vi "mixer.vi"(6 "Ready For Output":bool, 8 "Input Valid":bool, 9 "cos":fxp<+/-,16,2>, 10 "sin":fxp<+/-,16,2>, 11 "AI":fxp<+/-,16,1>) -> (0 "Output Valid":bool, 2 "Y":fxp<+/-,20,2> format="%.19g", 3 "X":fxp<+/-,20,2> format="%.19g", 4 "Ready For Input":bool=TRUE)   [LabVIEW 2018, in "SCTL.lvlib"]
doc: "This VI is used in four wire handshake."
uses:
  SCTL.lvlib
  <vilib>/rvi/FXPMathLib/FxpMul/XNode/nifxpmath_Multiplier.xnode
  <vilib>/rvi/FXPMathLib/sim/FxpSim.dll
panel:
  # "Inputs"
  # "Outputs"
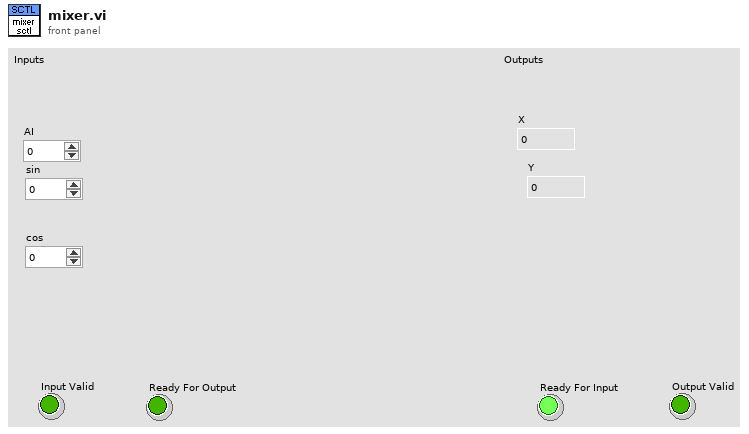
[diagram p1: front panel]
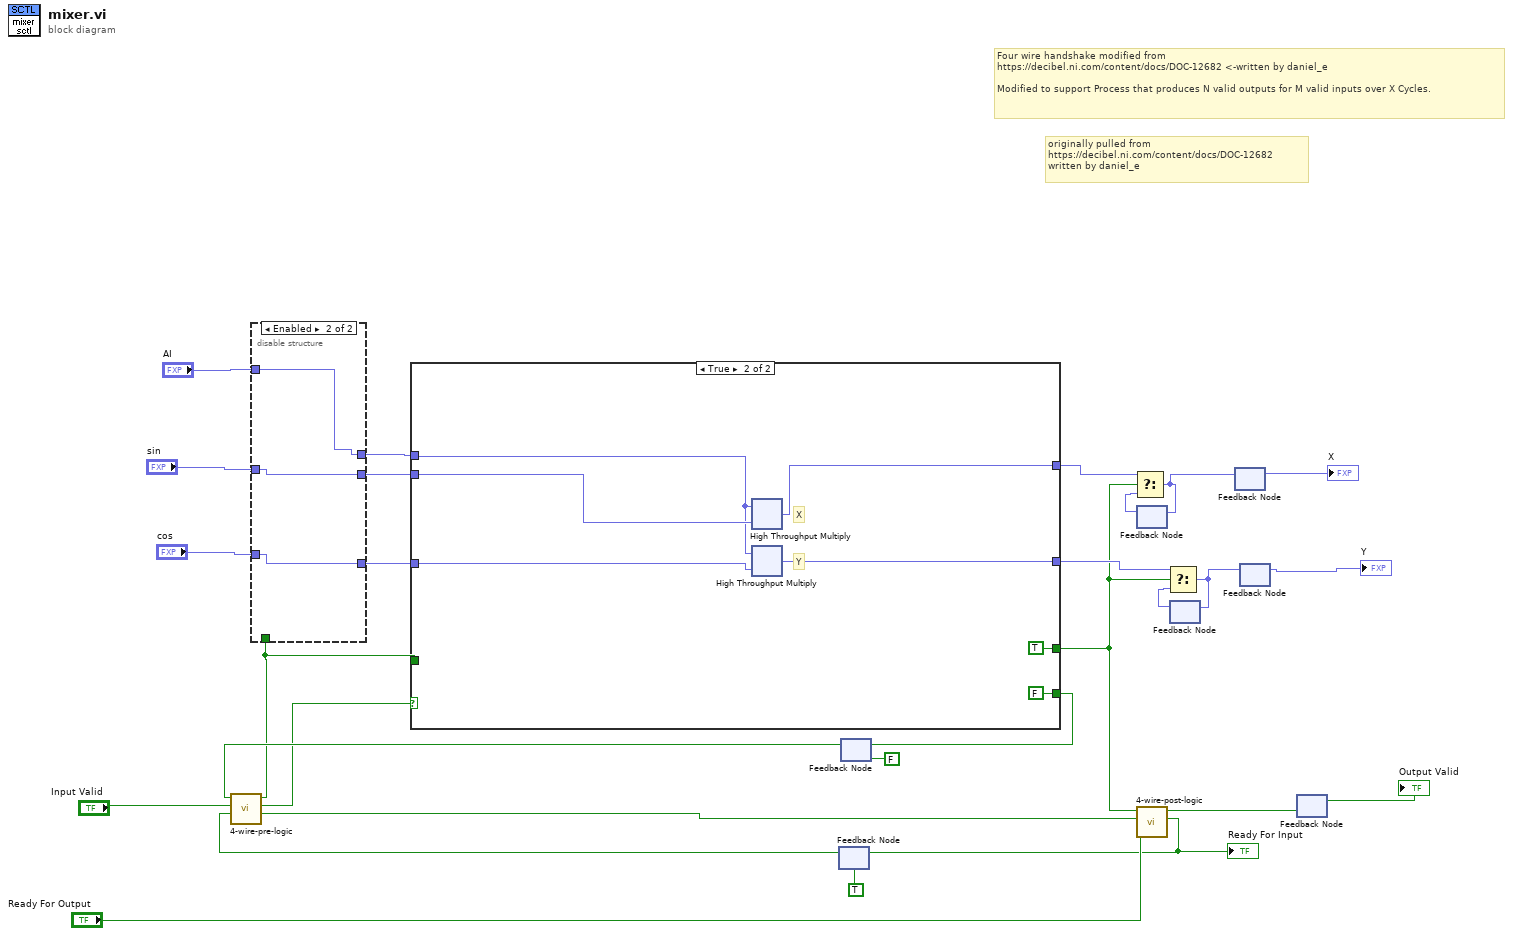
[diagram p0: block diagram]
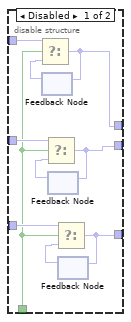
[diagram p2: hidden frame]
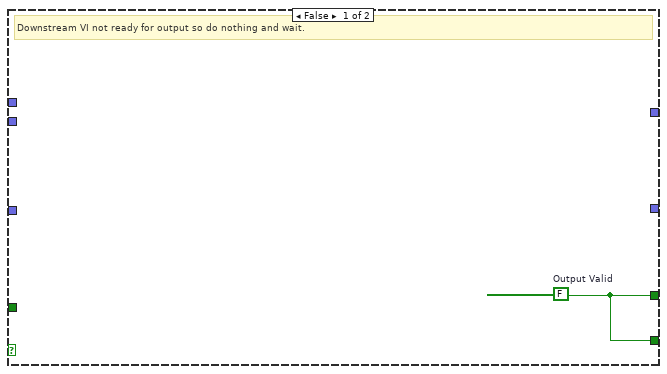
[diagram p3: hidden frame]
diagram:
  # "originally pulled from \nhttps://decibel.ni.com/content/docs/DOC-12682\nwritten by daniel_e"
  # "Four wire handshake modified from \nhttps://decibel.ni.com/content/docs/DOC-12682 <-written by daniel_e\n\nModified to support Process that produces N valid outputs for M valid inputs over X Cycles."
  n1 = feedback #1(TRUE ("x .and. y?")) -> (w25:bool)
  n2 = feedback #2(FALSE ("x .and. y?")) -> (w23:bool)
  n3 = call "4-wire-pre-logic.vi"("ready for input in"=w25, "Input Valid in"="Input Valid", "needs more iter in"=w23) -> ("register state out"=w27:bool, "excecute"=w22:bool, "buffer input!"=w10:bool)  [unwired: 6 in]
  n4 = disable-structure shown="Enabled" {
    disable-tunnel: "AI" -> [w36 w41]
    disable-tunnel: [w35 w41] -> w16
    disable-tunnel: "sin" -> [w34 w40]
    disable-tunnel: [w33 w40] -> w14
    disable-tunnel: "cos" -> [w31 w39]
    disable-tunnel: [w30 w39] -> w12
    disable-tunnel: w10 -> [w29 _]
    frame Disabled {
      n5 = feedback #3() -> (w38:fxp<+/-,16,1>)  [unwired: 1 in]
      n6 = Select(t=w36, s=w29, f=w38) -> (s? t:f=w35:fxp<+/-,16,1>)
      n7 = feedback-in #3(w35) -> ()
      n8 = feedback #4() -> (w37:fxp<+/-,16,2>)  [unwired: 1 in]
      n9 = Select(t=w34, s=w29, f=w37) -> (s? t:f=w33:fxp<+/-,16,2>)
      n10 = feedback-in #4(w33) -> ()
      n11 = feedback #5() -> (w32:fxp<+/-,16,2>)  [unwired: 1 in]
      n12 = Select(t=w31, s=w29, f=w32) -> (s? t:f=w30:fxp<+/-,16,2>)
      n13 = feedback-in #5(w30) -> ()
    }
    frame Enabled {
    }
  }
  n14 = case shown="True" w22 {
    tunnel: [w42 TRUE ("Output Valid")] -> w8
    tunnel: w10 -> [_ _]
    tunnel: [w42 FALSE ("Output Valid")] -> w21
    tunnel: w16 -> [_ w45]
    tunnel: w14 -> [_ w47]
    tunnel: w12 -> [_ w46]
    tunnel: [_ w44] -> w11
    tunnel: [_ w43] -> w9
    frame False {
      w42 = FALSE  # Output Valid
      # "Downstream VI not ready for output so do nothing and wait."
    }
    frame True {
      # "Y"
      # "X"
      n15 = xnode ("High Throughput Multiply")("x"=w45, "y"=w47) -> ("x*y"=w44:fxp<+/-,20,2>)
      n16 = xnode ("High Throughput Multiply")("x"=w45, "y"=w46) -> ("x*y"=w43:fxp<+/-,20,2>)
    }
  }
  n17 = feedback-in #2(w21) -> ()
  n18 = feedback #6() -> (w2:fxp<+/-,20,2>)  [unwired: 1 in]
  n19 = Select(t=w11, s=w8, f=w2) -> (s? t:f=w26:fxp<+/-,20,2>)
  n20 = feedback-in #6(w26) -> ()
  n21 = call "4-wire-post-logic.vi"("Ready For Output in"="Ready For Output", "register state in"=w27, "output valid in"=w8) -> ("ready for input out"=w18:bool, "output valid out"=w4:bool)  [unwired: 7 in]
  "Ready For Input" <- w18
  n22 = feedback-in #1(w18) -> ()
  n23 = feedback #7() -> (w1:fxp<+/-,20,2>)  [unwired: 1 in]
  n24 = Select(t=w9, s=w8, f=w1) -> (s? t:f=w6:fxp<+/-,20,2>)
  n25 = feedback-in #7(w6) -> ()
  n26 = feedback-in #8(w26) -> ()
  n27 = feedback #8() -> (→"X":fxp<+/-,20,2>)  [unwired: 1 in]
  n28 = feedback #9() -> (→"Y":fxp<+/-,20,2>)  [unwired: 1 in]
  n29 = feedback-in #9(w6) -> ()
  n30 = feedback #10() -> (→"Output Valid":bool)  [unwired: 1 in]
  n31 = feedback-in #10(w4) -> ()
